vi "MDAQ_IndexIncNew.vi"(10 "Input Cluster":T1) -> (2 "Output Cluster":T1)   [LabVIEW 2021]
uses:
  FunctionVIS/GUI_Def.ctl
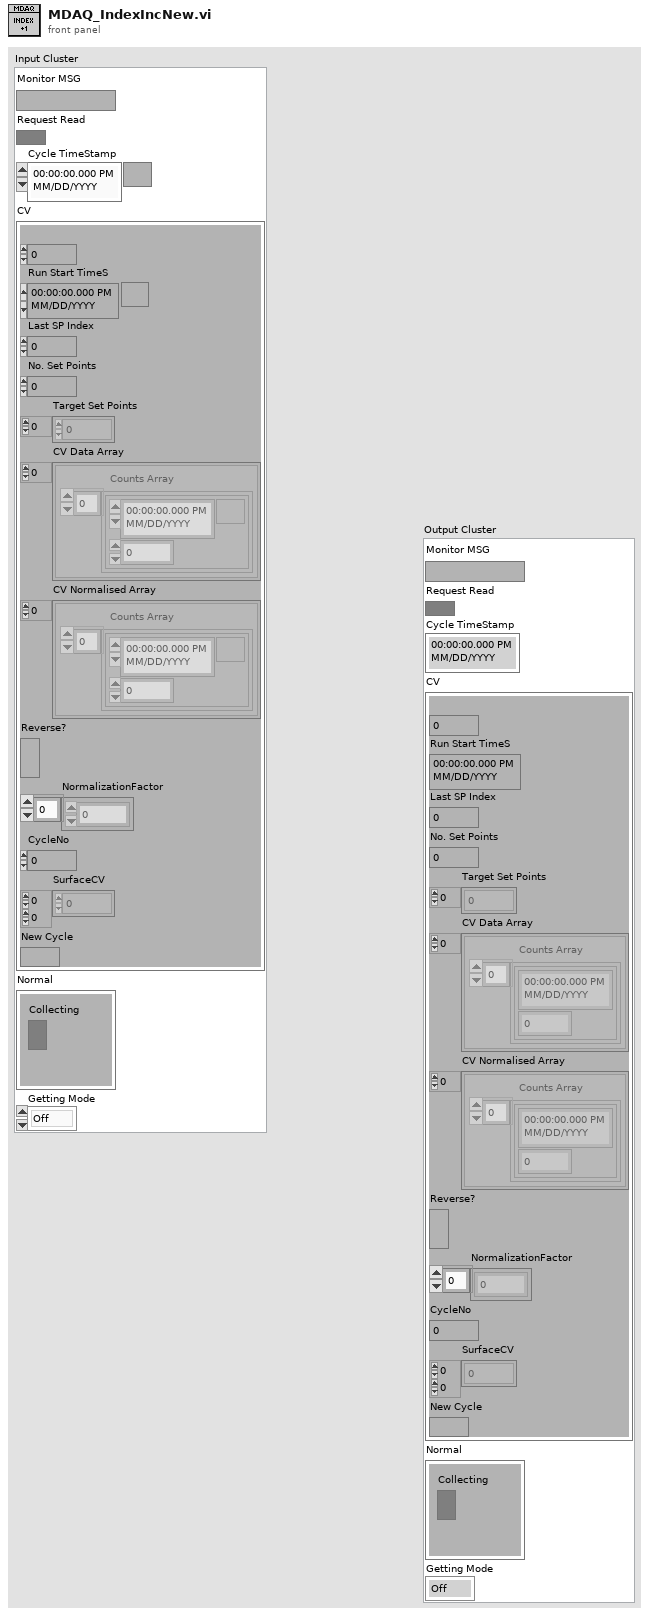
[diagram p1: front panel]
types:
  T1 = typedef "GUI_Def.ctl" = cluster{"Monitor MSG":string, "Request Read":bool, "Cycle TimeStamp":timestamp, "CV":cluster{"Set Point Index":u32, "Run Start TimeS":timestamp, "Last SP Index":u32, "No. Set Points":u32, "Target Set Points":dbl[], "CV Data Array":cluster{"Counts Array":cluster{timestamp, i32}[]}[], "CV Normalised Array":cluster{"Counts Array":cluster{timestamp, dbl}[]}[], "Reverse?":bool, "NormalizationFactor":i32[], "CycleNo":i32, "SurfaceCV":dbl[][], "New Cycle":bool}, "Normal":cluster{"Collecting":bool}, "Getting Mode":enum16{"Off", "Normal", "CV"}}
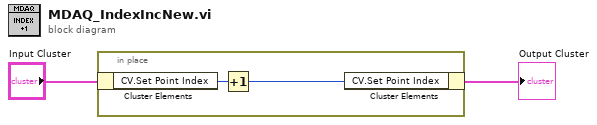
[diagram p0: block diagram]
diagram:
  n1 = in-place {
    n2 = in-place-cluster #1("Input Cluster") -> ("CV.Set Point Index"=w4:u32)
    n3 = Increment(x=w4) -> (x+1=w3:u32)
    n4 = in-place-cluster #1("CV.Set Point Index"=w3) -> (→"Output Cluster":T1)
  }
